vi "Subvi pixel clock generator old.vi"   [LabVIEW 2017]
uses:
  <vilib>/Platform/TimedLoop/XDataNode/timing_clust.ctl
  <vilib>/Platform/TimedLoop/XDataNode/nitl_modes.ctl
  <vilib>/Platform/TimedLoop/XDataNode/wakeup.ctl
  <vilib>/rvi/Emulation/niFpgaGetClockAttributes.vi
  <vilib>/rvi/Emulation/niFpgaSctlEmulationGetInTimedLoop.vi
  <vilib>/rvi/Emulation/niFpgaEmulationReportErrorSimple.vi
  <vilib>/rvi/Emulation/niFpgaCriticalErrorInLSC.vi
  Detector/GV line clock change.vi
  <vilib>/rvi/Emulation/niFpgaProcessEmulError.vi
  <vilib>/rvi/eio/common/nirviEmuTemplateMethod_errors.vi
  <vilib>/Platform/TimedLoop/XDataNode/XDataNode.xnode
  <vilib>/eio/EIONode/EIONode.xnode
  <vilib>/Platform/TimedLoop/XDataNode/XDNodeRunTimeDep.lvlib
types:
  T1 = typedef "XDNodeRunTimeDep.lvlib/timing_clust.ctl" = cluster{"Expected End [f-1]":u64, "Actual End [f-1]":u64, "Finished Late? [f-1]":bool, "Expected End [i-1]":u64, "Actual End [i-1]":u64, "Finished Late? [i-1]":bool, "Expected Start [i]":u64, "Actual Start [i]":u64, "Expected Start [f]":u64, "Actual Start [f]":u64, "Source Name":string, "Structure Name":string, "Period":i64, "Deadline":i64, "Offset":i64, "Start":i64, "Priority":i32, "Timeout":i32, "Mode":T2, "Wakeup Reason":T3, "Error":errorcluster, "Source Type":string, "Secondary Source Type":string, "Global End Time":u64, "Global Start Time":u64, "Frame Duration":u64, "Iteration Duration":u64, "Assigned CPU":i32, "I/O Scan Engine Mode":u32}
  T2 = typedef "XDNodeRunTimeDep.lvlib/nitl_modes.ctl" = enum32{"No Change", "Process missed periods, maintain original phase", "Discard missed periods, maintain original phase", "Process missed periods, ignore original phase", "Discard missed periods, ignore original phase"}
  T3 = typedef "XDNodeRunTimeDep.lvlib/wakeup.ctl" = enum32{"Normal", "Aborted", "Asynchronous wakeup", "Timing source error", "Timed loop error", "Timeout"}
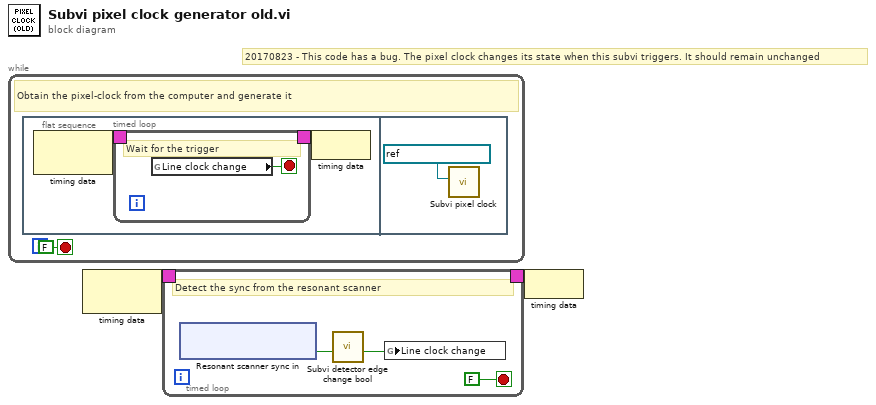
[diagram p0: block diagram]
diagram:
  # "20170823 - This code has a bug. The pixel clock changes its state when this subvi triggers. It should remain unchanged"
  n1 = while {
    stop <- FALSE stop-if-true
    # "Obtain the pixel-clock from the computer and generate it"
    n2 = flat-sequence {
      frame #0 {
        n3 = node-c288() -> (w5:T1)  [unwired: 1 in]
        n4 = timed-loop {
          timing: w5 -> [_]
          timing-out: [_] -> w4
          stop <- w6 stop-if-true
          # "Wait for the trigger"
          n5 = global read "GV line clock change.vi" "Line clock change"() -> (w6:bool)
        }
        n6 = node-c288(w4) -> ()
      }
      frame #1 {
        n7 = call "Subvi pixel clock.vi"("Memory label"=refnum<k21> "Pixel clock buffer") -> ()  [unwired: 11 in]
      }
    }
  }
  n8 = node-c288() -> (w2:T1)  [unwired: 1 in]
  n9 = timed-loop {
    timing: w2 -> [_]
    timing-out: [_] -> w1
    stop <- FALSE stop-if-true
    # "Detect the sync from the resonant scanner"
    n10 = xnode "Resonant scanner sync in"() -> ("Connector0/DIO0"=w13:bool)  [unwired: 1 in, 1 out]
    n11 = call "Subvi detector edge change bool.vi"("Input"=w13) -> ("Output"=w12:bool)  [unwired: 8 in]
    n12 = global write "GV line clock change.vi" "Line clock change"(w12) -> ()
  }
  n13 = node-c288(w1) -> ()
